vi "TSM DAQmx Relay Close Sessions.vi"(0 "TSM context":T1) -> (15 "error out":errorcluster)   [LabVIEW 2019]
doc: "Use this VI to reset and close all sessions for all NI-RELAY (Switch) instruments in the Semiconductor Module Context."
uses:
  <vilib>/NI_TestStand_SemiconductorModule/NI_TestStand_Semiconductor_Module.lvlibp/PinMap/General/SemiconductorModuleContext.ctl
  <vilib>/NI_TestStand_SemiconductorModule/NI_TestStand_Semiconductor_Module.lvlibp
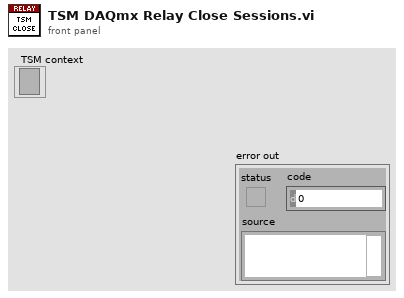
[diagram p1: front panel]
types:
  T1 = typedef "NI_TestStand_Semiconductor_Module.lvlibp/SemiconductorModuleContext.ctl" = refnum<k7>
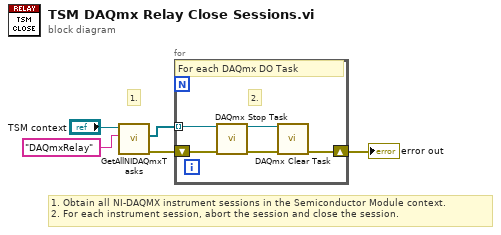
[diagram p0: block diagram]
diagram:
  # "1. Obtain all NI-DAQMX instrument sessions in the Semiconductor Module context.\n2. For each instrument session, abort the session and close the session."
  # "1."
  n1 = call <vilib>:"GetAllNIDAQmxTasks.vi"("Task Type"="DAQmxRelay", "Semiconductor Module Context"="TSM context") -> ("error out"=w4:errorcluster, "DAQmx Tasks"=w5:refnum<k21>[])  [unwired: 7 in, 1 out]
  n2 = for {
    tunnel: w5 -> [w9] mode=indexing
    shift-right: [w7] -> w1
    shift-left: w4 -> [w10]
    # "2."
    # "For each DAQmx DO Task"
    n3 = call <vilib>:"DAQmx Stop Task.vi"("task/channels in"=w9, "error in"=w10) -> ("task out"=w8:refnum<k21>, "error out"=w6:errorcluster)  [unwired: 12 in]
    n4 = call <vilib>:"DAQmx Clear Task.vi"("task in"=w8, "error in"=w6) -> ("error out"=w7:errorcluster)  [unwired: 13 in]
  }
  "error out" <- w1
